vi "Test Rotate.vi"(8 "error in (no error)":errorcluster, 11 "Instrument.Cryostat in":refnum<class "Instrument.Cryostat.lvclass">) -> (0 "error out":errorcluster, 3 "Instrument.Cryostat out":refnum<class "Instrument.Cryostat.lvclass">)   [LabVIEW 2016, in "Instrument.Cryostat.lvclass"]
uses:
  Instrument.Cryostat.lvclass
  <vilib>/addons/_JKI Toolkits/Caraya/classes/Assert/Assert.lvclass
  <vilib>/addons/_JKI Toolkits/Caraya/classes/Test/Test.lvclass
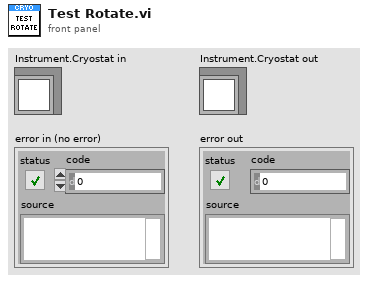
[diagram p1: front panel]
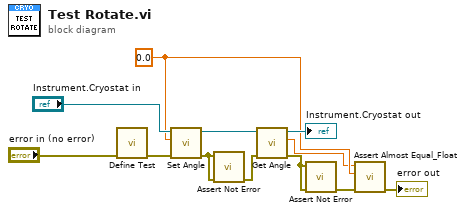
[diagram p0: block diagram]
diagram:
  w4 = 0.0 ("Angle (°)")
  n1 = call <vilib>:"Define Test.vi"("error in (no error)"="error in (no error)") -> ("error out"=w1:errorcluster)  [unwired: 10 in]
  n2 = call-dynamic "Set Angle.vi"("error in (no error)"=w1, "Angle (°)"=w4, "Instrument.Cryostat in"="Instrument.Cryostat in") -> ("error out"=w9:errorcluster, "Instrument.Cryostat out"=w5:refnum<class "Instrument.Cryostat.lvclass">)  [unwired: 7 in]
  n3 = call <vilib>:"Assert Not Error.vi"("error in (no error)"=w9, "Not Error?"=w9) -> ("error out"=w10:errorcluster)  [unwired: 9 in]
  n4 = call-dynamic "Get Angle.vi"("error in (no error)"=w10, "Instrument.Cryostat in"=w5) -> ("error out"=w11:errorcluster, "Angle (°)"=w3:dbl, "Instrument.Cryostat out"=→"Instrument.Cryostat out":refnum<class "Instrument.Cryostat.lvclass">)  [unwired: 7 in]
  n5 = call <vilib>:"Assert Not Error.vi"("error in (no error)"=w11, "Not Error?"=w11) -> ("error out"=w12:errorcluster)  [unwired: 9 in]
  n6 = call <vilib>:"Assert Almost Equal_Float.vi"("error in (no error)"=w12, "Y"=w4, "X"=w3) -> ("error out"=→"error out":errorcluster)  [unwired: 8 in]
